vi "Curtin1_ReadWriteFRFGraphData.vi"(8 "Type":T3 items=["FRF", "rad phase unwrapped", "deg phase unwrapped", "rad phase wrapped", "deg phase wrapped", "White Plots", "MJ Map", "Real and Imaginary"], 9 "FRF":refnum<vi>, 11 "Task":enum16{"Read", "Save"}(ring)) -> (0 "y log?":bool, 1 "x log?":bool, 2 "dB":dbl)   [LabVIEW 2022 SP3]
uses:
  GraphType.ctl
  <vilib>/Utility/miscctls.llb/LVRangeTypeDef.ctl
  Mic/Mic_Global.vi
panel:
  out "Graph settings":T2
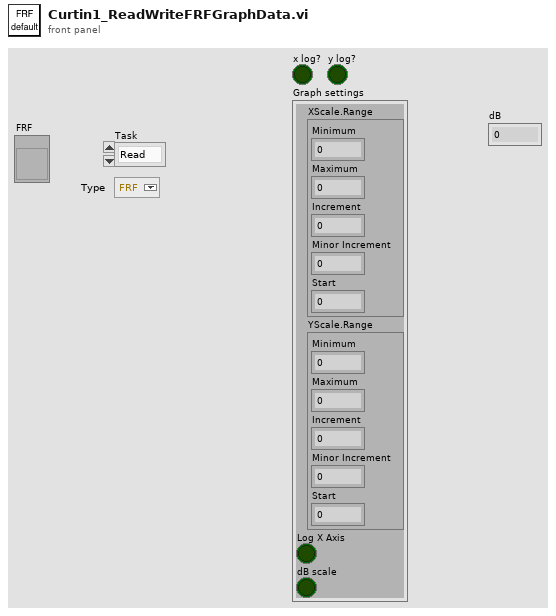
[diagram p1: front panel]
types:
  T1 = typedef "LVRangeTypeDef.ctl" = cluster{"Minimum":dbl, "Maximum":dbl, "Increment":dbl, "Minor Increment":dbl, "Start":dbl}
  T2 = cluster{"XScale.Range":T1, "YScale.Range":T1, "Log X Axis":bool, "dB scale":bool}
  T3 = typedef "GraphType.ctl" = u16
  T4 = cluster{"Alerts":bool, "Log X Axis":bool, "dB scale":bool, "Averaging":bool, "Fade":dbl, "Centroids?":bool}
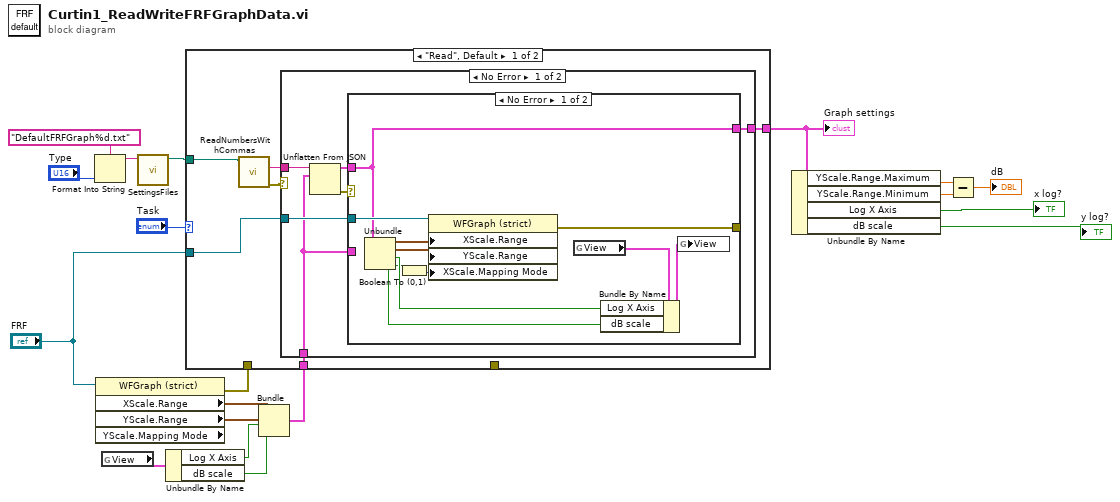
[diagram p0: block diagram]
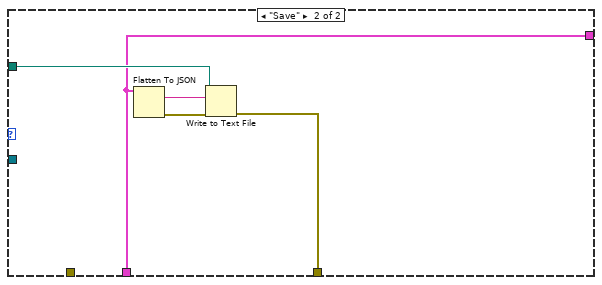
[diagram p4: hidden frame]
diagram:
  n1 = Format Into String(format string="DefaultFRFGraph%d.txt" ("name or relative path"), "Type") -> (resulting string=w2:string)  [unwired: 2 in, 1 out]
  n2 = property class="WFGraph (strict)" props=["XScale", "Range", "YScale", "Range", "YScale", "Mapping Mode"](reference="FRF") -> (error out=w14:errorcluster, "XScale.Range"=w18:T1, "YScale.Range"=w17:T1)  [unwired: 1 in, 2 out]
  n3 = global read "Mic_Global.vi" "View"() -> (w7:T4)
  n4 = call "SettingsFiles.vi"("settings file name"=w2) -> ("file path"=w1:path)  [unwired: 9 in, 1 out]
  n5 = Unbundle By Name(w7) -> ("Log X Axis"=w6:bool, "dB scale"=w5:bool)
  n6 = Bundle("XScale.Range"=w18, "YScale.Range"=w17, "Log X Axis"=w6, "dB scale"=w5) -> (w16:T2)  [unwired: 1 in]
  n7 = case shown="\"Read\", Default" "Task" {
    tunnel: w1 -> [w22 w46]
    tunnel: [_ w45] -> _
    tunnel: w16 -> [w25 w44]
    tunnel: "FRF" -> [w24 _]
    tunnel: w14 -> [_ _]
    tunnel: [w23 w44] -> w13
    frame "Read", Default {
      n8 = call "ReadNumbersWithCommas.vi"("file (use dialog)"=w22) -> ("error out"=w21:errorcluster, "text"=w20:string)  [unwired: 7 in, 2 out]
      n9 = case shown="No Error" w21 {
        tunnel: w20 -> [w31 _]
        tunnel: w25 -> [w26 w43]
        tunnel: w24 -> [w28 _]
        tunnel: [w27 w43] -> w23
        frame No Error {
          n10 = Unflatten From JSON(JSON string=w31, type and defaults=w26) -> (value=w29:T2, error out=w30:errorcluster)  [unwired: 5 in]
          n11 = case shown="No Error" w30 {
            tunnel: w29 -> [w37 _]
            tunnel: w28 -> [w41 _]
            tunnel: [w38 _] -> _
            tunnel: [w37 w42] -> w27
            tunnel: w26 -> [_ w42]
            frame No Error {
              n12 = Unbundle(w37) -> ("XScale.Range"=w40:T1, "YScale.Range"=w39:T1, "Log X Axis"=w34:bool, "dB scale"=w33:bool)
              n13 = Boolean To (0,1)(Boolean=w33) -> (0, 1=w32:i16)
              n14 = property class="WFGraph (strict)"(reference=w41, "XScale.Range"=w40, "YScale.Range"=w39, "XScale.Mapping Mode"=w32) -> (error out=w38:errorcluster)  [unwired: 1 in, 1 out]
              n15 = global read "Mic_Global.vi" "View"() -> (w36:T4)
              n16 = Bundle By Name(cluster=w36, "Log X Axis"=w34, "dB scale"=w33) -> (w35:T4)
              n17 = global write "Mic_Global.vi" "View"(w35) -> ()
            }
            frame Error {
            }
          }
        }
        frame Error {
        }
      }
    }
    frame "Save" {
      n18 = Flatten To JSON(anything=w44) -> (JSON string=w48:string, 11:w47:errorcluster)  [unwired: 2 in]
      n19 = Write to Text File(file (use dialog)=w46, text=w48, error in=w47) -> (error out=w45:errorcluster)  [unwired: 1 in, 2 out]
    }
  }
  "Graph settings" <- w13
  n20 = Unbundle By Name(w13) -> ("YScale.Range.Maximum"=w11:dbl, "YScale.Range.Minimum"=w12:dbl, "Log X Axis"=→"x log?":bool, "dB scale"=→"y log?":bool)
  n21 = Subtract(x=w11, y=w12) -> (x-y=→"dB":dbl)
